vi "CDW_SpecPage.vi"(10 "Spec Page Interface":T1, 11 "MetaDataObj in":refnum<class "MetaDataObj.lvclass">) -> (3 "MetaDataObj out":refnum<class "MetaDataObj.lvclass">)   [LabVIEW 2014, in "NIVS_ScriptedModuleTemplate_MetaDataObj.lvclass"]
uses:
  NIVS_ScriptedModuleTemplate_MetaDataObj.lvclass
  <vilib>/Utility/sysdir.llb/System Directory Type.ctl
  TypDef/CD Wizard - Execution Mode.ctl
  <resource>/dialog/NewProjectWizard/Spec Page Interface.ctl
  <resource>/dialog/NewProjectWizard/MetaDataObj/MetaDataObj.lvclass
panel:
  in  "Custom Device Name":string
  in  "Custom Device Path":path
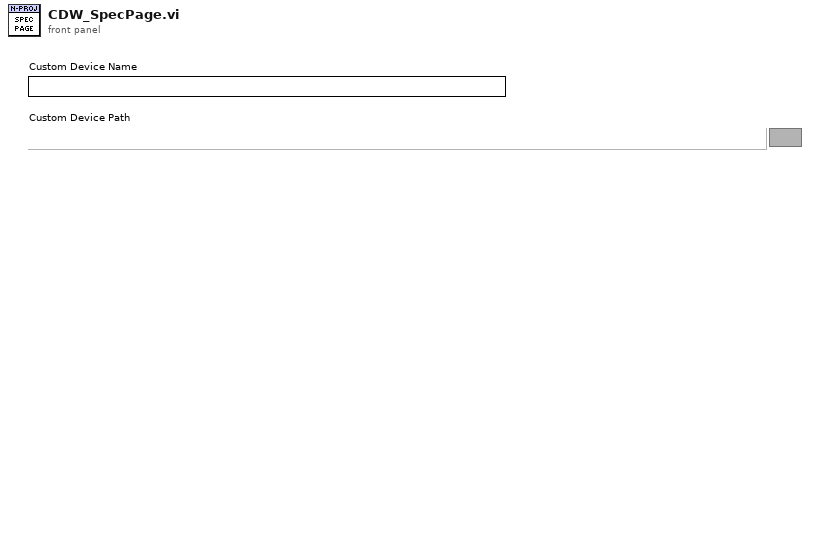
[diagram p1: front panel]
types:
  T1 = typedef "Spec Page Interface.ctl" = cluster{"\"Tab Forward To\" Refnum":refnum<vi>, "\"Tab Backward To\" Refnum":refnum<vi>, "Errors":refnum<user-event>, "Quit":refnum<user-event>}
  T2 = typedef "CD Wizard - Execution Mode.ctl" = enum16{"Asynchronous", "Inline HW Interface", "Inline Model Interface", "Inline Timing and Sync", "Asynchronous Timing and Sync"}
  T3 = typedef "System Directory Type.ctl" = i32
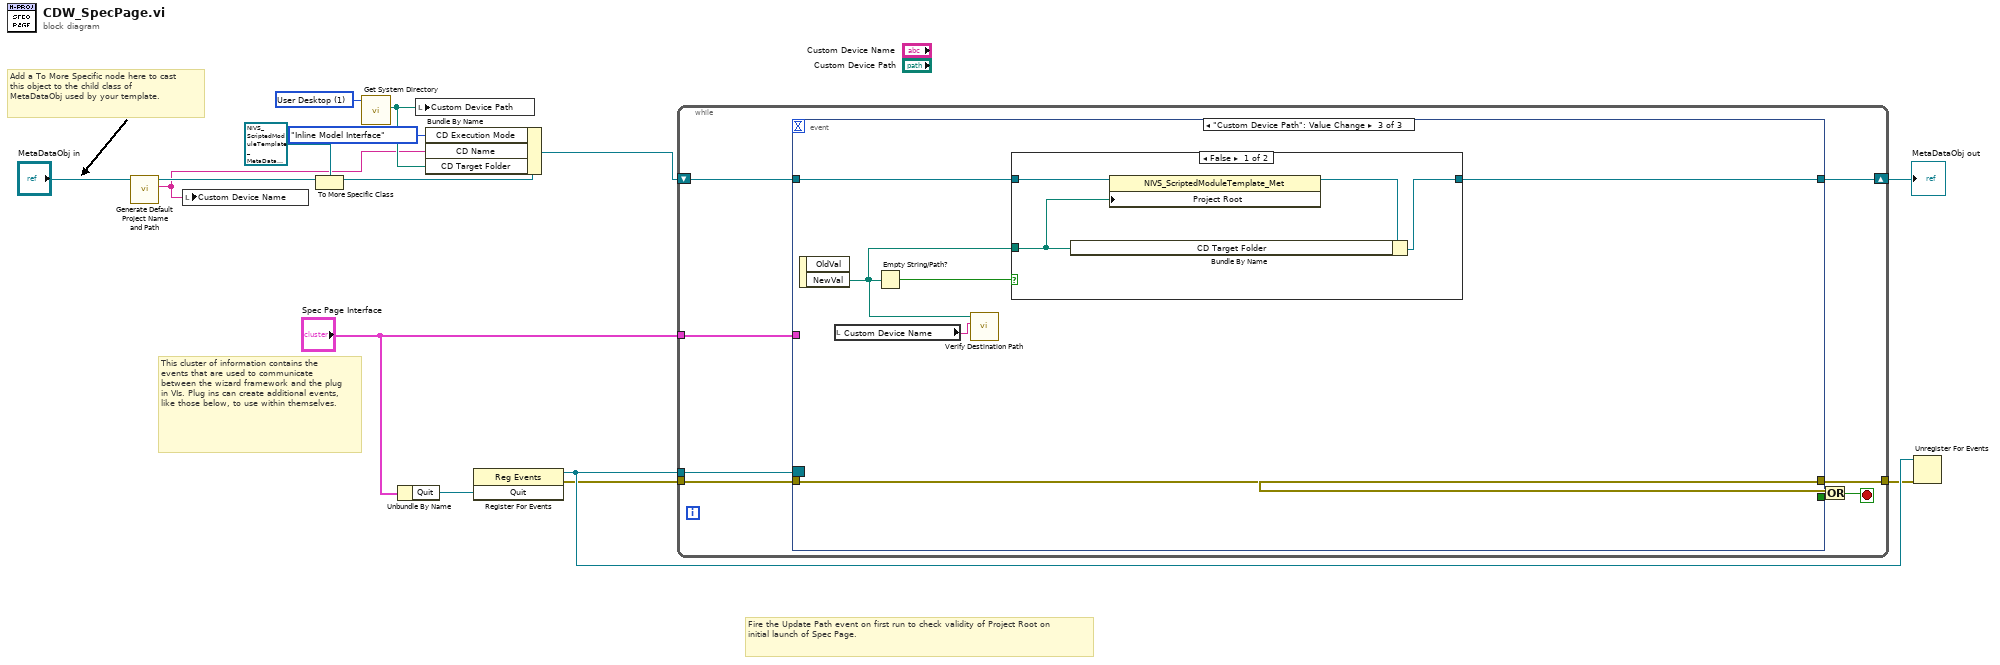
[diagram p0: block diagram]
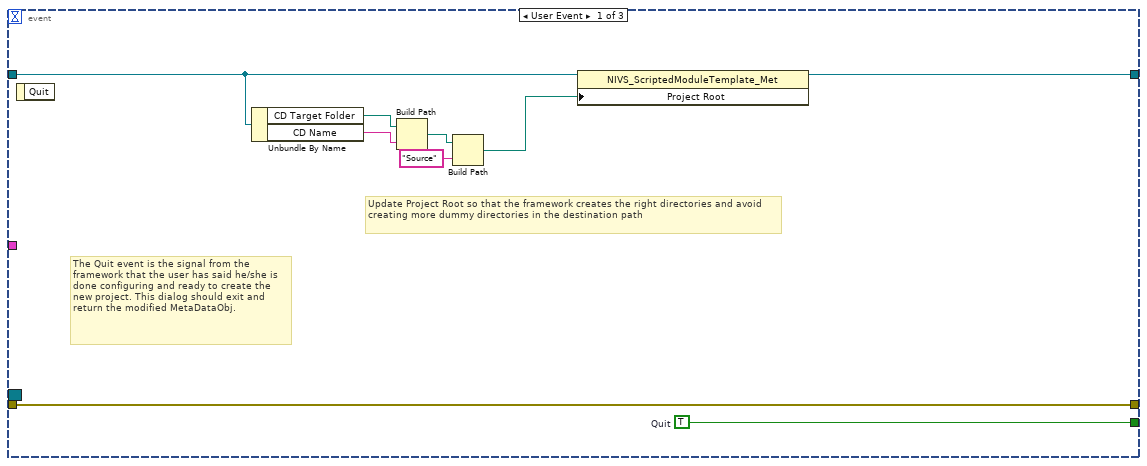
[diagram p2: hidden frame]
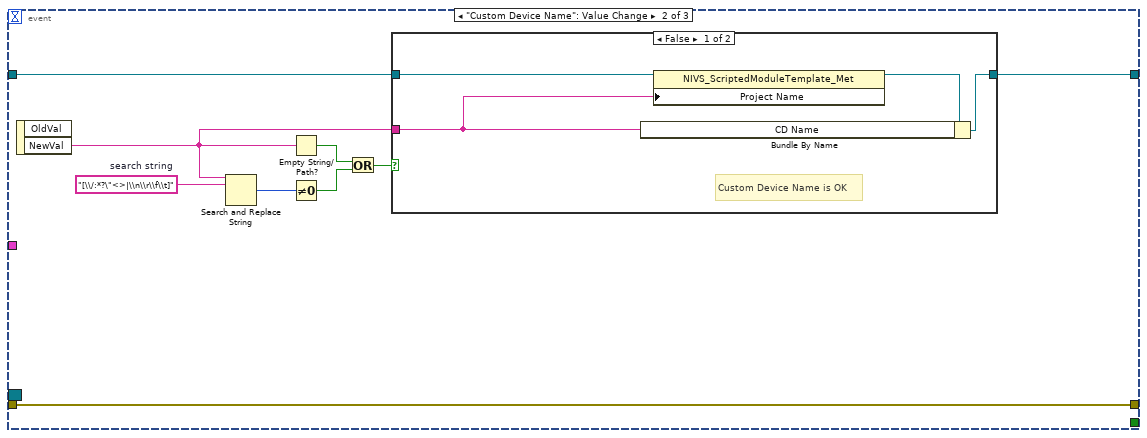
[diagram p3: hidden frame]
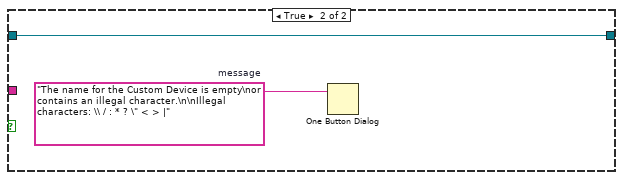
[diagram p4: hidden frame]
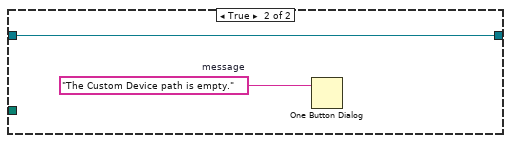
[diagram p5: hidden frame]
diagram:
  w6 = T3 1 items=["User Home"=0, "User Desktop"=1, "User Documents"=2, "User Application Data"=3, "User Preferences"=4, "User Temporary"=5, "Public Documents"=6, "Public Application Data"=7, "Public Preferences"=8, "Public Cache"=13, "System Core Libraries"=9, "System Installed Libraries"=10, "Application Files"=11, "Boot Volume Root"=12] ("system directory type")
  # "Fire the Update Path event on first run to check validity of Project Root on initial launch of Spec Page."
  # "This cluster of information contains the events that are used to communicate between the wizard framework and the plug in VIs. Plug ins can create additional events, like those below, to use within themselves."
  # "Add a To More Specific node here to cast this object to the child class of MetaDataObj used by your template."
  n1 = call <resource>:"Generate Default Project Name and Path.vi"("DNL_MetaDataObj in"="MetaDataObj in") -> ("Project Name"=w3:string, "DNL_MetaDataObj out"=w8:refnum<class "MetaDataObj.lvclass">)  [unwired: 8 in, 1 out]
  n2 = local write "Custom Device Name"(w3) -> ()
  n3 = To More Specific Class(target class=refnum<class "NIVS_ScriptedModuleTemplate_MetaDataObj.lvclass"> refnum ("NIVS_CDW_MetaDataObj.lvclass"), reference=w8) -> (specific class reference=w5:refnum<class "NIVS_ScriptedModuleTemplate_MetaDataObj.lvclass">)  [unwired: 1 in, 1 out]
  n4 = call <vilib>:"Get System Directory.vi"("system directory type"=w6) -> ("system directory"=w4:path)  [unwired: 10 in]
  n5 = Unbundle By Name("Spec Page Interface") -> ("Quit"=w15:refnum<user-event>)
  n6 = local write "Custom Device Path"(w4) -> ()
  n7 = Bundle By Name(cluster=w5, "CD Execution Mode"=CD_Wizard_-_Execution_Mode."Inline Model Interface" ("CD Wizard - Internal Data.Common Information.CD Execution Mode"), "CD Name"=w3, "CD Target Folder"=w4) -> (w2:refnum<class "NIVS_ScriptedModuleTemplate_MetaDataObj.lvclass">)
  n8 = register-events(w15) -> (reference out=w14:refnum<event-registration>, error out=w9:errorcluster)  [unwired: 2 in]
  n9 = while {
    tunnel: "Spec Page Interface" -> [w21]
    shift-right: [w20] -> w11
    shift-left: w2 -> [w19]
    tunnel: w14 -> [w23]
    tunnel: w9 -> [w22]
    tunnel: [w16] -> w12
    stop <- w18 stop-if-true
    n10 = event shown="[2] \"Custom Device Path\": Value Change" {
      selector: w23 -> [_ _ _]
      dyn-events: _ -> [_ _ _]
      timeout: _ -> [_ _ _]
      tunnel: w21 -> [_ _ _]
      tunnel: [w32 _ _] -> w17
      tunnel: [w31 w41 w53] -> w16
      tunnel: w22 -> [w31 w41 w53]
      tunnel: [w30 w35 w50] -> w20
      tunnel: w19 -> [w29 w33 w51]
      event User Event {
        w32 = TRUE  # Quit
        # "Update Project Root so that the framework creates the right directories and avoid creating more dummy directories in the destination path"
        # "The Quit event is the signal from the framework that the user has said he/she is done configuring and ready to create the new project. This dialog should exit and return the modified MetaDataObj."
        n11 = event-data() -> ()  [unwired: 1 in, 1 out]
        n12 = Unbundle By Name(w29) -> ("CD Target Folder"=w28:path, "CD Name"=w24:string)
        n13 = Build Path(base path=w28, name or relative path=w24) -> (appended path=w27:path)
        n14 = Build Path(base path=w27, name or relative path="Source") -> (appended path=w25:path)
        n15 = property class="NIVS_ScriptedModuleTemplate_Met"(reference=w29, "Project Root"=w25) -> (reference out=w30:refnum<class "NIVS_ScriptedModuleTemplate_MetaDataObj.lvclass">)  [unwired: 1 in, 1 out]
      }
      event "Custom Device Name": Value Change {
        w37 = "[\\/:*?\"<>|\\n\\r\\f\\t]"  # search string
        n16 = event-data() -> ("NewVal"=w34:string)  [unwired: 1 in, 1 out]
        n17 = Search and Replace String(input string=w34, search string=w37) -> (number of replacements=w38:i32)  [unwired: 6 in, 3 out]
        n18 = Empty String/Path?(string/path=w34) -> (empty?=w39:bool)
        n19 = Not Equal To 0?(x=w38) -> (x != 0?=w40:bool)
        n20 = Or(x=w39, y=w40) -> (x .or. y?=w36:bool)
        n21 = case shown="False" w36 {
          tunnel: w33 -> [w44 w46]
          tunnel: [w45 w46] -> w35
          tunnel: w34 -> [w42 _]
          frame False {
            # "Custom Device Name is OK"
            n22 = property class="NIVS_ScriptedModuleTemplate_Met"(reference=w44, "Project Name"=w42) -> (reference out=w43:refnum<class "NIVS_ScriptedModuleTemplate_MetaDataObj.lvclass">)  [unwired: 1 in, 1 out]
            n23 = Bundle By Name(cluster=w43, "CD Name"=w42) -> (w45:refnum<class "NIVS_ScriptedModuleTemplate_MetaDataObj.lvclass">)
          }
          frame True {
            w47 = "The name for the Custom Device is empty\nor contains an illegal character.\n\nIllegal characters: \\ / : * ? \" < > |"  # message
            n24 = One Button Dialog(message=w47) -> ()  [unwired: 1 in, 1 out]
          }
        }
      }
      event "Custom Device Path": Value Change {
        n25 = event-data() -> ("NewVal"=w49:path)  [unwired: 1 in, 1 out]
        n26 = local read "Custom Device Name"() -> (w48:string)
        n27 = Empty String/Path?(string/path=w49) -> (empty?=w52:bool)
        n28 = call "Verify Destination Path.vi"("Custom Device Name"=w48, "Custom Device Path"=w49) -> ()  [unwired: 9 in, 1 out]
        n29 = case shown="False" w52 {
          tunnel: w51 -> [w56 w58]
          tunnel: [w57 w58] -> w50
          tunnel: w49 -> [w54 _]
          frame False {
            n30 = property class="NIVS_ScriptedModuleTemplate_Met"(reference=w56, "Project Root"=w54) -> (reference out=w55:refnum<class "NIVS_ScriptedModuleTemplate_MetaDataObj.lvclass">)  [unwired: 1 in, 1 out]
            n31 = Bundle By Name(cluster=w55, "CD Target Folder"=w54) -> (w57:refnum<class "NIVS_ScriptedModuleTemplate_MetaDataObj.lvclass">)
          }
          frame True {
            w59 = "The Custom Device path is empty."  # message
            n32 = One Button Dialog(message=w59) -> ()  [unwired: 1 in, 1 out]
          }
        }
      }
    }
    n33 = Or(x=w16, y=w17) -> (x .or. y?=w18:bool)
  }
  "MetaDataObj out" <- w11
  n34 = Unregister For Events(event registration refnum=w14, error in=w12) -> ()  [unwired: 1 out]
